vi "Broadcast Item Received Status Update.vi"(8 "error in (no error)":errorcluster, 11 "Customer in":refnum<class "Customer.lvclass">) -> (0 "error out":errorcluster, 3 "Customer out":refnum<class "Customer.lvclass">)   [LabVIEW 2020, in "Customer.lvclass"]
uses:
  Customer.lvclass
  C:/Users/anton/Documents/GitHub/Triarc-Examples/Coffee Shop/Person/Person.lvclass
  Customer.lvclass/Customer.ctl
  Person/Person.lvclass
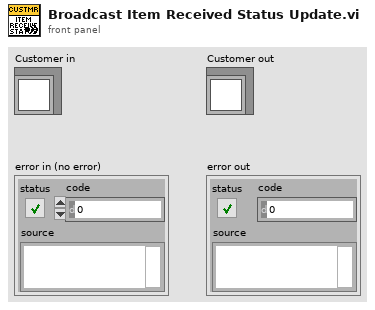
[diagram p1: front panel]
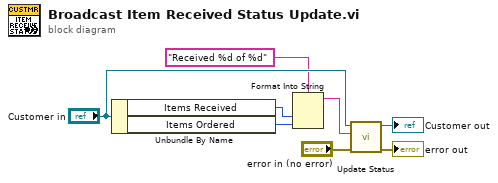
[diagram p0: block diagram]
diagram:
  n1 = Unbundle By Name("Customer in") -> ("Items Received"=w3:u32, "Items Ordered"=w4:u32)
  n2 = Format Into String(format string="Received %d of %d", w3, w4) -> (resulting string=w8:string)  [unwired: 2 in, 1 out]
  n3 = call "Update Status.vi"("error in (no error)"="error in (no error)", "Status"=w8, "Person In"="Customer in") -> ("error out"=→"error out":errorcluster, "Person Out"=→"Customer out":refnum<class "Customer.lvclass">)  [unwired: 7 in]
